vi "MotorMultiInfo.vi"(3 "Names":string[](array[string]), 10 "error in (no error)":errorcluster) -> (0 "Names out":string[](array[string]), 2 "Axis status":T1(array[cluster]), 6 "error out":errorcluster)   [LabVIEW 2009]
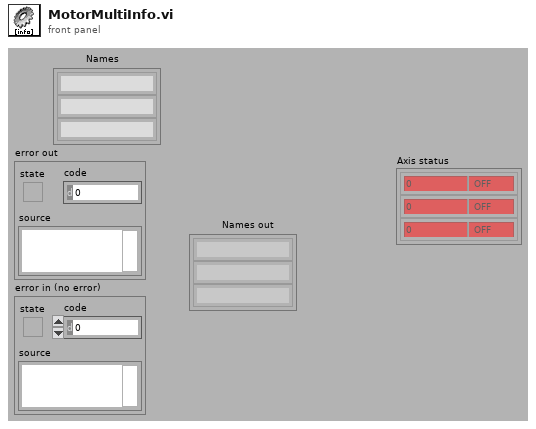
[diagram p1: front panel]
types:
  T1 = cluster{"Managed?":bool, "Status":enum16{"OFF", "IDLE", "MOVING", "HOMING"}, "Position":i32}[]
  T2 = cluster{"Managed?":bool, "Status":enum16{"OFF", "IDLE", "MOVING", "HOMING"}, "Position":i32}
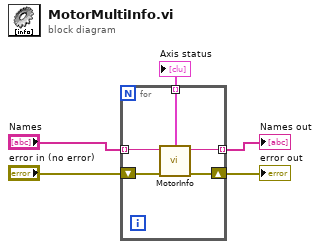
[diagram p0: block diagram]
diagram:
  n1 = for {
    shift-right: [w9] -> w5
    shift-left: "error in (no error)" -> [w10]
    tunnel: "Names" -> [w8] mode=indexing
    tunnel: [w7] -> w2 mode=indexing
    tunnel: [w6] -> w1 mode=indexing
    n2 = call "MotorInfo.vi"("Motor"=w8, "error in (no error)"=w10) -> ("Motor out"=w7:string, "Axis status"=w6:T2, "error out"=w9:errorcluster)  [unwired: 5 in]
  }
  "error out" <- w5
  "Names out" <- w2
  "Axis status" <- w1
